vi "Set DAQ Analog Data Value.vi"(0 "DAQ":refnum<class "DAQ.lvclass">, 5 "IOName (enum)":variant, 7 "Value":dbl, 9 "Name":string, 11 "error in (no error)":errorcluster) -> (4 "DAQ":refnum<class "DAQ.lvclass">, 8 "Value out":dbl, 15 "error out":errorcluster)   [LabVIEW 2017, in "DAQ.lvclass"]
doc: "Developed by Kevin Thompson\nkevin@thompsonengineering.net\n\nCopyright 2018-2020\nThompson Engineering, LLC"
uses:
  DAQ.lvclass
  DAQ.lvclass/DAQ.ctl
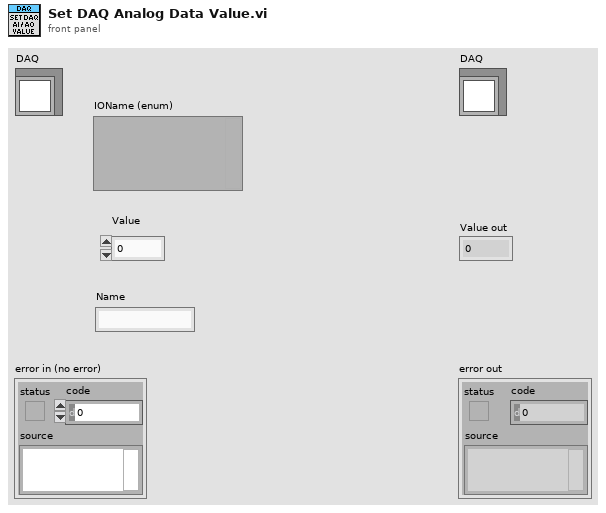
[diagram p1: front panel]
types:
  T1 = typedef "Type Descriptor Enumeration__ogtk.ctl" = enum8{"<Null>", "I8", "I16", "I32", "I64", "U8", "U16", "U32", "U64", "SGL", "DBL", "EXT", "CSG", "CDB", "CXT", "0x0F", "0x10", "0x11", "0x12", "0x13", "0x14", "Enum U8", "Enum U16", "Enum U32", "Enum U64", "SGL PQ", "DBL PQ", "EXT PQ", "CSG PQ", "CDB PQ", "CXT PQ", "0x1F", "0x20", "Boolean", "0x22", "0x23", "0x24", "0x25", "0x26", "0x27", "0x28", "0x29", "0x2A", "0x2B", "0x2C", "0x2D", "0x2E", "0x2F", "String", "0x31", "Path", "Pict", "0x34", "0x35", "0x36", "DAQ", "0x38", "0x39", "0x3A", "0x3B", "0x3C", "0x3D", "0x3E", "0x3F", "Array", "0x41", "0x42", "0x43", "0x44", "0x45", "0x46", "0x47", "0x48", "0x49", "0x4A", "0x4B", "0x4C", "0x4D", "0x4E", "0x4F", "Cluster", "0x51", "0x52", "Variant", "Waveform", "0x55", "0x56", "0x57", "0x58", "0x59", "0x5A", "0x5B", "0x5C", "0x5D", "0x5E", "0x5F", "0x60", "0x61", "0x62", "0x63", "0x64", "0x65", "0x66", "0x67", "0x68", "0x69", "0x6A", "0x6B", "0x6C", "0x6D", "0x6E", "0x6F", "Refnum"}
  T2 = typedef "TD Dynamic CVT DVR--ref.ctl" = refnum<data-value>
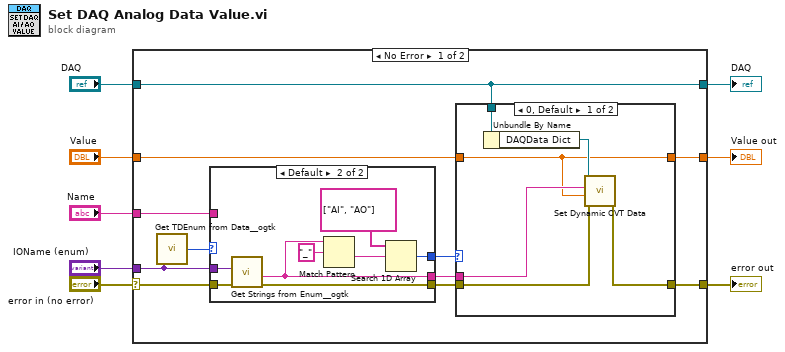
[diagram p0: block diagram]
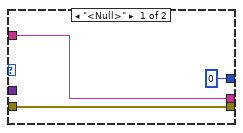
[diagram p2: hidden frame]
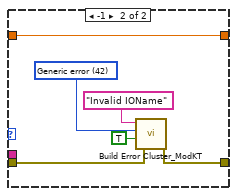
[diagram p3: hidden frame]
diagram:
  n1 = case shown="No Error" "error in (no error)" {
    selector: "error in (no error)" -> [w19 w45]
    tunnel: [w15 w45] -> w7
    tunnel: [w18 w44] -> w5
    tunnel: "DAQ" -> [w18 w44]
    tunnel: "IOName (enum)" -> [w11 _]
    tunnel: [w12 w43] -> w3
    tunnel: "Value" -> [w16 w43]
    tunnel: "Name" -> [w9 _]
    frame No Error {
      n2 = call <userlib>:"Get TDEnum from Data__ogtk.vi"("Data"=w11) -> ("Type Descriptor Enumeration"=w10:T1)  [unwired: 4 in]
      n3 = case shown="Default" w10 {
        tunnel: w11 -> [_ w30]
        tunnel: w19 -> [w21 w29]
        tunnel: [w21 w28] -> w17
        tunnel: [0 ("index of element") w24] -> w14
        tunnel: [w22 w23] -> w13
        tunnel: w9 -> [w22 _]
        frame "<Null>" {
        }
        frame Default {
          n4 = call <userlib>:"Get Strings from Enum__ogtk.vi"("error in (no error)"=w29, "Enum"=w30) -> ("error out"=w28:errorcluster, "String Value"=w23:string)  [unwired: 6 in, 2 out]
          n5 = Match Pattern(string=w23, regular expression="_") -> (after substring=w26:string)  [unwired: 1 in, 3 out]
          n6 = Search 1D Array(1D array=string[] ["AI", "AO"], element=w26) -> (index of element=w24:i32)  [unwired: 1 in]
        }
      }
      n7 = case shown="0, Default" w14 {
        tunnel: w18 -> [w36 _]
        tunnel: w13 -> [w34 _]
        tunnel: w17 -> [w33 w38]
        tunnel: w16 -> [w31 w42]
        tunnel: [w32 w37] -> w15
        tunnel: [w31 w42] -> w12
        frame 0, Default {
          n8 = Unbundle By Name(w36) -> ("DAQData Dict"=w35:T2)
          n9 = call <vilib>:"Set Dynamic CVT Data.vi"("error in (no error)"=w33, "value"=w31, "DataName"=w34, "dCVT DVR"=w35) -> ("error out"=w32:errorcluster)  [unwired: 5 in, 2 out]
        }
        frame -1 {
          w40 = 42 items=["No error", "Argument error", "Memory is full", "Out of zone", "End of file", "File already open", "Generic file I/O error", "File not found", "File permission error", "Disk is full", "Duplicate path", "Too many files open", "System feature not enabled", "Resource file not found", "Cannot add resource", "Resource not found", "Image not found", "Image memory error", "Pen does not exist", "Config type invalid", "Config token not found", "Config parse error", "Config memory error", "Bad external code format", "Bad external code offset", "External code not present", "Null window", "Destroy window error", "Null menu", "Print aborted", "Bad print record", "Print driver error", "Windows error during printing", "Memory error during printing", "Print dialog error", "Generic print error", "Invalid device refnum", "Device not found", "Device parameter error", "Device unit error", "Cannot open device", "Device call aborted", "Generic error", "Cancelled by user", "Object ID too low", "Object ID too high", "Object not in heap", "Unknown heap", "Unknown object (invalid DefProc)", "Unknown object (DefProc not in table)", "Message out of range", "Invalid (null) method", "Unknown message", "Manager call not supported", "Bad address", "Network operation in progress", "Network operation timed out", "Connection is busy", "Network attribute not supported", "Network error", "Address in use", "System out of memory", "Connection aborted", "Connection refused", "Not connected", "Already connected", "Connection closed", "Initialization error (interapplication manager)", "Bad occurrence", "Wait on unbound occurrence handler", "Occurrence queue overflow", "Datalog type conflict", "Unused", "Unrecognized type (interapplication manager)", "Memory corrupt", "Failed to make temporary DLL", "Old CIN version", "Drag socket not found", "Failed to load drop-object", "Failed to register OLE object", "Failed to release OLE object", "Format specifier type mismatch", "Unknown format specifier", "Too few format specifiers", "Too many format specifiers", "Scan failed", "Newer CIN version", "Error converting to variant", "Runtime menu error", "Password tampered", "Variant attribute not found", "Incompatible variant data type", "Event data is not available", "Event Store is not present", "Occurrence is not found", "Event Queue is not created", "Event info is not available", "Refnum passed is NULL", "Error retrieving Class GUID", "Error retrieving CoClass GUID", "Error retrieving TypeLib GUID.", "Bad built application magic bytes.", "Specific driver is different from the specific driver associated with the Logical Name.", "There is no session opened to the class driver.", "Max Error", "MAX - Error with config objects", "MAX - Error loading configuration", "MAX - Group not supported"]
          n10 = call <vilib>:"Build Error Cluster_ModKT .vi"("Prepend String (\"\")"="Invalid IOName" ("Prepend String (\"\")"), "code"=w40, "error? (F)"=TRUE, "error in (no error)"=w38) -> ("error out"=w37:errorcluster)  [unwired: 3 in, 1 out]
        }
      }
    }
    frame Error {
    }
  }
  "error out" <- w7
  "DAQ" <- w5
  "Value out" <- w3
